vi "PTScanner.set step values.vi"(0 "i ref in":refnum<vi>, 5 "error in(no error)":errorcluster) -> (14 "i ref out":refnum<vi>, 19 "error out":errorcluster)   [LabVIEW 2014, in "PTScanner.lvlib"]
uses:
  PTScanner.lvlib
  CS_Core/CSSystem/CSSystemLib/CSSystemLib.lvlib
  CS_Core/BaseProcess/BaseProcess.lvlib
  _common/PTUtils/PTUtils.lvlib
  CSlibraries-extern/DimLVEvent/LVDimInterface/LVDimInterface.lvlib
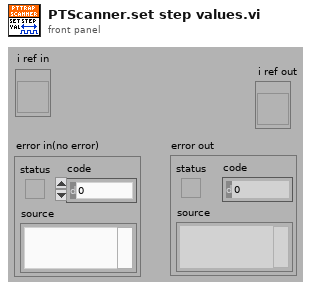
[diagram p1: front panel]
types:
  T1 = typedef "PTScanner.lvlib/PTScanner.i attribute.ctl" = cluster{"Object cmds":T2[], "Steps":cluster{"Finished":bool, "cmd setup":T3[]}[], "curStep":i32, "DIM IDs":cluster{"AllFinished":i32, "Finished":i32, "curStep":i32, "nofSteps":i32, "NomValues":i32[], "1D-Min":i32, "1D-Max":i32, "Dimensions":i32, "MaxDimensions":i32, "ScanedDeviceNames":i32[]}, "All Finished":bool, "DIMs in use":string[], "Running":bool, "Scan Delay":u32, "loop":bool, "Paused":bool, "Formed":bool}
  T2 = typedef "PTScanner.lvlib/PTScanner.obj parameters.ctl" = cluster{"object":string, "DIM address":string, "method":string, "data descriptor":string, "method parameters":cluster{"Name":string, "Descr":string, "Value":string, "Value?":bool}[], "Call Mode":enum16{"Simple DIM", "Synchronous"}, "actValue":dbl, "Centroid":dbl, "Minus Delta":dbl, "Plus Delta":dbl, "increment":dbl, "DIM Status":cluster{"no link":bool, "quality":i32, "Time Stamp":timestamp}, "range":dbl, "DIMChannelIndex":i32}
  T3 = typedef "PTScanner.lvlib/PTScanner.step obj parameters.ctl" = cluster{"obj index":i32, "nomValue":dbl, "fulfilled":bool}
  T4 = cluster{"Name":string, "Descr":string, "Value":string, "Value?":bool}[]
  T5 = typedef "CoreDefs.rawDataType.ctl" = i8[]
  T6 = typedef "CoreDefs.call_type.ctl" = cluster{"Object":string, "Selector":string, "CallType":enum16{"simple", "synchronous", "asynchronous"}, "Async Object":string, "Async Selector":string, "Data Descriptor":T7, "Data":T5, "Error #":i32, "Expire":u32}
  T7 = typedef "BaseProcess.lvlib/BaseProcess.descriptor string definition.ctl" = string
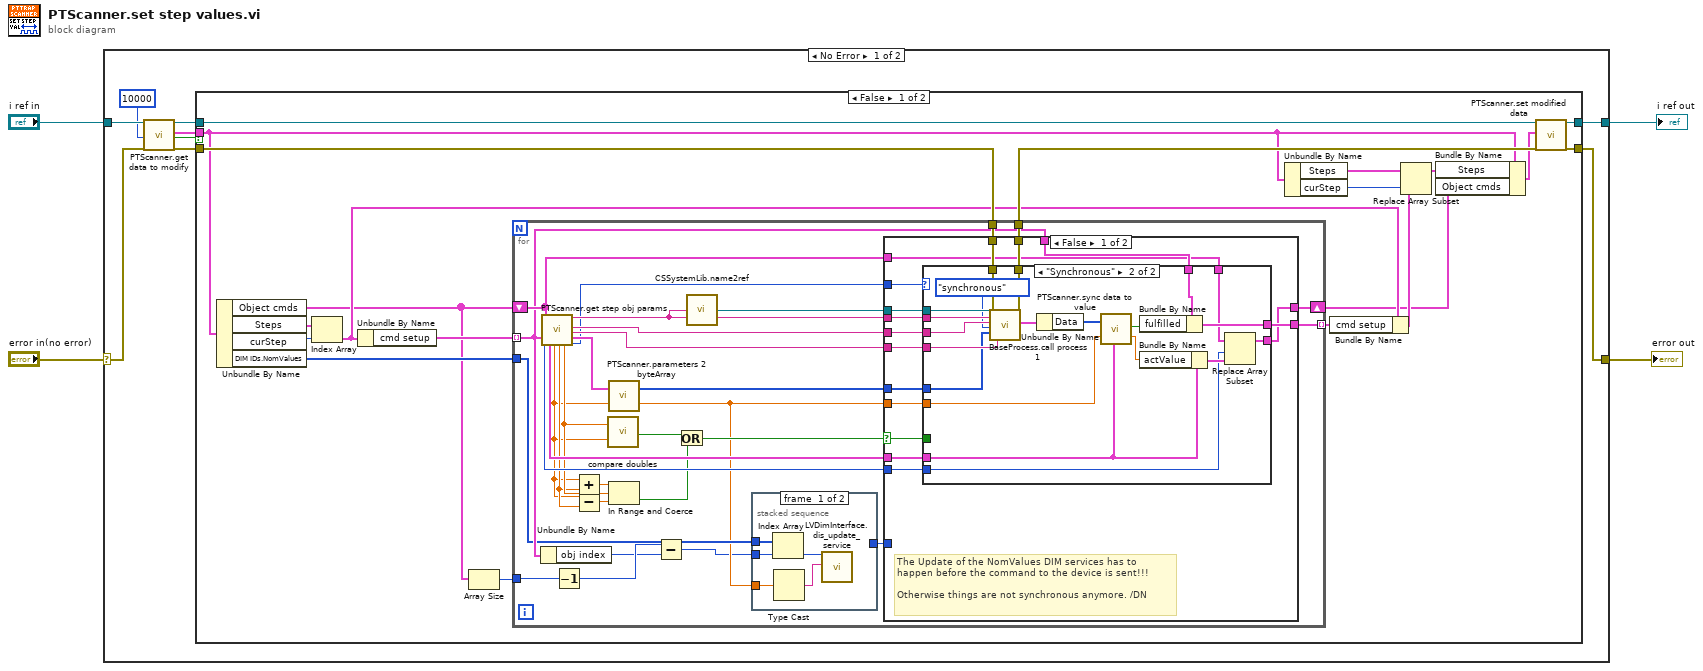
[diagram p0: block diagram]
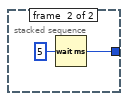
[diagram p2: hidden frame]
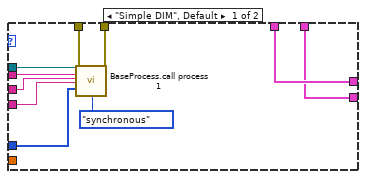
[diagram p3: hidden frame]
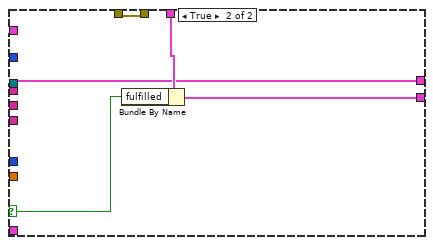
[diagram p4: hidden frame]
diagram:
  n1 = case shown="No Error" "error in(no error)" {
    selector: "error in(no error)" -> [w13 w123]
    tunnel: [w6 w123] -> w3
    tunnel: [w9 w124] -> w2
    tunnel: "i ref in" -> [w12 w124]
    frame No Error {
      n2 = call "PTScanner.get data to modify.vi"("i ref in"=w12, "ms timeout (10000)"=10000, "error in (no error)"=w13) -> ("i ref out"=w10:refnum<vi>, "i attribute"=w5:T1, "timed out"=w8:bool, "error out"=w11:errorcluster)  [unwired: 13 in]
      n3 = case shown="False" w8 {
        tunnel: w11 -> [w33 w122]
        tunnel: w10 -> [w32 w121]
        tunnel: [w31 w121] -> w9
        tunnel: [w30 w122] -> w6
        tunnel: w5 -> [w22 _]
        frame False {
          n4 = Unbundle By Name(w22) -> ("Object cmds"=w14:T2[], "Steps"=w28:cluster{"Finished":bool, "cmd setup":T3[]}[], "curStep"=w29:i32, "DIM IDs.NomValues"=w17:i32[])
          n5 = Index Array(array=w28, index=w29) -> (element=w21:cluster{"Finished":bool, "cmd setup":T3[]})
          n6 = Unbundle By Name(w21) -> ("cmd setup"=w16:T3[])
          n7 = Array Size(array=w14) -> (size(s)=w15:i32)
          n8 = for {
            tunnel: w16 -> [w41] mode=indexing
            tunnel: w33 -> [w62]
            tunnel: [w60] -> w27
            tunnel: [w54] -> w19 mode=indexing
            shift-right: [w51] -> w18
            shift-left: w14 -> [w52]
            tunnel: w17 -> [w40]
            tunnel: w15 -> [w37]
            n9 = Unbundle By Name(w41) -> ("obj index"=w34:i32)
            n10 = call "PTScanner.get step obj params.vi"("Objects"=w52, "step object params"=w41) -> ("obj index"=w50:i32, "obj params"=w53:T2, "nomValue"=w39:dbl, "range"=w43:dbl, "actValue"=w49:dbl, "Object"=w58:string, "Set value method"=w56:string, "Data descriptor"=w57:string, "Method Input Parameters"=w55:T4, "Call Mode"=w42:enum16{"Simple DIM", "Synchronous"})  [unwired: 3 in, 5 out]
            n11 = Decrement(x=w37) -> (x-1=w35:i32)
            n12 = Add(x=w39, y=w43) -> (x+y=w44:dbl)
            n13 = Subtract(x=w39, y=w43) -> (x-y=w45:dbl)
            n14 = call "compare doubles.vi"("base value"=w49, "value to compare"=w39) -> ("Equal"=w48:bool)  [unwired: 17 in]
            n15 = call "PTScanner.parameters 2 byteArray.vi"("Parameters"=w55, "nomValue"=w39) -> ("byteArray out"=w59:T5)  [unwired: 17 in]
            n16 = In Range and Coerce(upper limit=w44, x=w49, lower limit=w45) -> (In Range?=w46:bool)  [unwired: 1 out]
            n17 = Subtract(x=w35, y=w34) -> (x-y=w36:i32)
            n18 = Or(x=w48, y=w46) -> (x .or. y?=w47:bool)
            n19 = call "CSSystemLib.name2ref.vi"("name"=w58) -> ("obj refnum"=w61:refnum<vi>)
            n20 = stacked-sequence {
              tunnel: w40 -> [w63 _]
              tunnel: w36 -> [w67 _]
              tunnel: w39 -> [w64 _]
              tunnel: [_ w68] -> w38
              frame #0 {
                n21 = Index Array(array=w63, index=w67) -> (element=w66:i32)
                n22 = Type Cast(x=w64) -> (*(type *) &x=w65:string)  [unwired: 1 in]
                n23 = call "LVDimInterface.dis_update_service.vi"("my_serviceID"=w66, "data"=w65) -> ()  [unwired: 15 in, 3 out]
              }
              frame #1 {
                n24 = Wait (ms)(milliseconds to wait=u32 5) -> (millisecond timer value=w68:u32)
              }
            }
            n25 = case shown="False" w47 {
              selector: w47 -> [w78 w117]
              tunnel: w56 -> [w85 _]
              tunnel: w58 -> [w84 _]
              tunnel: w57 -> [w83 _]
              tunnel: w62 -> [w82 w120]
              tunnel: w61 -> [w81 _]
              tunnel: [w80 w120] -> w60
              tunnel: w59 -> [w79 _]
              tunnel: w39 -> [w70 _]
              tunnel: w41 -> [w77 w118]
              tunnel: [w76 w119] -> w54
              tunnel: w53 -> [w75 _]
              tunnel: w52 -> [w74 w116]
              tunnel: [w73 w116] -> w51
              tunnel: w50 -> [w72 _]
              tunnel: w42 -> [w71 _]
              tunnel: w38 -> [_ _]
              frame False {
                # "The Update of the NomValues DIM services has to \nhappen before the command to the device is sent!!!\n\nOtherwise things are not synchronous anymore. /DN"
                n26 = case shown="\"Synchronous\"" w71 {
                  tunnel: w85 -> [w91 w115]
                  tunnel: w84 -> [w92 w114]
                  tunnel: w83 -> [w90 w113]
                  tunnel: w82 -> [w89 w112]
                  tunnel: w81 -> [w93 w111]
                  tunnel: [w88 w110] -> w80
                  tunnel: w79 -> [w87 w107]
                  tunnel: w78 -> [_ _]
                  tunnel: w70 -> [_ w96]
                  tunnel: w77 -> [w95 w104]
                  tunnel: [w95 w103] -> w76
                  tunnel: w75 -> [_ w97]
                  tunnel: w74 -> [w94 w100]
                  tunnel: [w94 w99] -> w73
                  tunnel: w72 -> [_ w98]
                  frame "Simple DIM", Default {
                    n27 = call "BaseProcess.call process 1.vi"("i ref in"=w93, "Object"=w92, "Selector"=w91, "CallType"=enum16{"simple", "synchronous", "asynchronous"}."synchronous", "Data"=w87, "error in (no error)"=w89, "Data Descriptor"=w90) -> ("error out"=w88:errorcluster)  [unwired: 10 in, 2 out]
                  }
                  frame "Synchronous" {
                    n28 = call "BaseProcess.call process 1.vi"("i ref in"=w111, "Object"=w114, "Selector"=w115, "CallType"=enum16{"simple", "synchronous", "asynchronous"}."synchronous", "Data"=w107, "error in (no error)"=w112, "Data Descriptor"=w113) -> ("call cluster out"=w108:T6, "error out"=w110:errorcluster)  [unwired: 10 in, 1 out]
                    n29 = Unbundle By Name(w108) -> ("Data"=w106:T5)
                    n30 = call "PTScanner.sync data to value.vi"("byteArray"=w106, "nomValue"=w96, "obj params"=w97) -> ("matched"=w105:bool, "actValue"=w102:dbl)  [unwired: 15 in]
                    n31 = Bundle By Name(cluster=w104, "fulfilled"=w105) -> (w103:T3)
                    n32 = Bundle By Name(cluster=w97, "actValue"=w102) -> (w101:T2)
                    n33 = Replace Array Subset(array=w100, new element=w101, index=w98) -> (w99:T2[])
                  }
                }
              }
              frame True {
                n34 = Bundle By Name(cluster=w118, "fulfilled"=w117) -> (w119:T3)
              }
            }
          }
          n35 = Unbundle By Name(w22) -> ("Steps"=w24:cluster{"Finished":bool, "cmd setup":T3[]}[], "curStep"=w23:i32)
          n36 = Bundle By Name(cluster=w21, "cmd setup"=w19) -> (w20:cluster{"Finished":bool, "cmd setup":T3[]})
          n37 = Replace Array Subset(array=w24, new element=w20, index=w23) -> (w25:cluster{"Finished":bool, "cmd setup":T3[]}[])
          n38 = Bundle By Name(cluster=w22, "Steps"=w25, "Object cmds"=w18) -> (w26:T1)
          n39 = call "PTScanner.set modified data.vi"("i ref in"=w32, "CLASS.i attribute"=w26, "error in (no error)"=w27) -> ("i ref out"=w31:refnum<vi>, "error out"=w30:errorcluster)  [unwired: 15 in]
        }
        frame True {
        }
      }
    }
    frame Error {
    }
  }
  "error out" <- w3
  "i ref out" <- w2
